vi "Set Photon Counting Divisions.vi"(8 "error in (no error)":errorcluster, 10 "divisions":i32, 11 "noOfDivisions":u32) -> (0 "error out":errorcluster, 2 "divisions out":i32, 3 "function return":u32)   [LabVIEW 2014, in "atmcd32d.lvlib"]
doc: "unsigned int WINAPI SetPhotonCountingDivisions(at_u32 noOfDivisions, at_32 * divisions);"
uses:
  atmcd32d.lvlib
  atmcd32d.dll
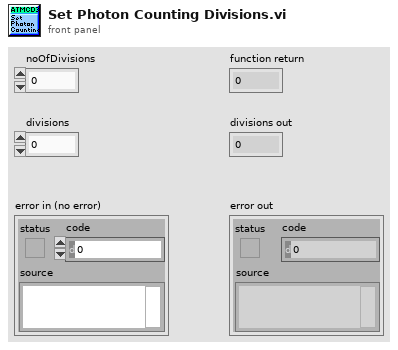
[diagram p1: front panel]
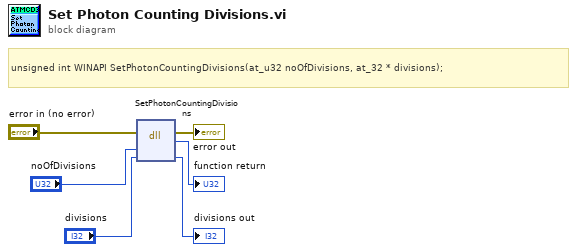
[diagram p0: block diagram]
diagram:
  # "unsigned int WINAPI SetPhotonCountingDivisions(at_u32 noOfDivisions, at_32 * divisions);"
  n1 = dll-call lib="C:/Users/Bakir/Documents/Lambda2-Testing/lib/Andorlib/atmcd32d.*" fn="SetPhotonCountingDivisions"(error in="error in (no error)", "noOfDivisions"="noOfDivisions", "divisions"="divisions") -> (error out=→"error out":errorcluster, →"function return":u32, "divisions"=→"divisions out":i32)  [unwired: 3 in, 1 out]
